vi "ThermoV_ControlSweep_NoMean_ExperimentalCode_AC_LV2017.vi"() -> ()   [LabVIEW 2017]
panel:
  in  "Operate HVpp\nOutput Timer":bool caption="Reset"
  out "modular 13":dbl
  in  "Number of seconds for \neach HVpp case state":dbl=30.0
  out "Elapsed Time (s)":dbl
  out "DC Value":dbl[](array[numeric]) format="%#.6f"
  in  "Saving Avg?":bool
  in  "Filename":path=path "trial_1.lvm"
  in  "STOP":bool
  in  "Save Waveform":bool
  out "Peak2Peak V":dbl[](array[numeric])
  out "Waveform Chart":dynamicdata(graph)
  # "AI 0:  Thermoelectric Voltage\nAI 1:  Heater Current (Voltage)\n\nAO 0:  Applied Heater Voltage"
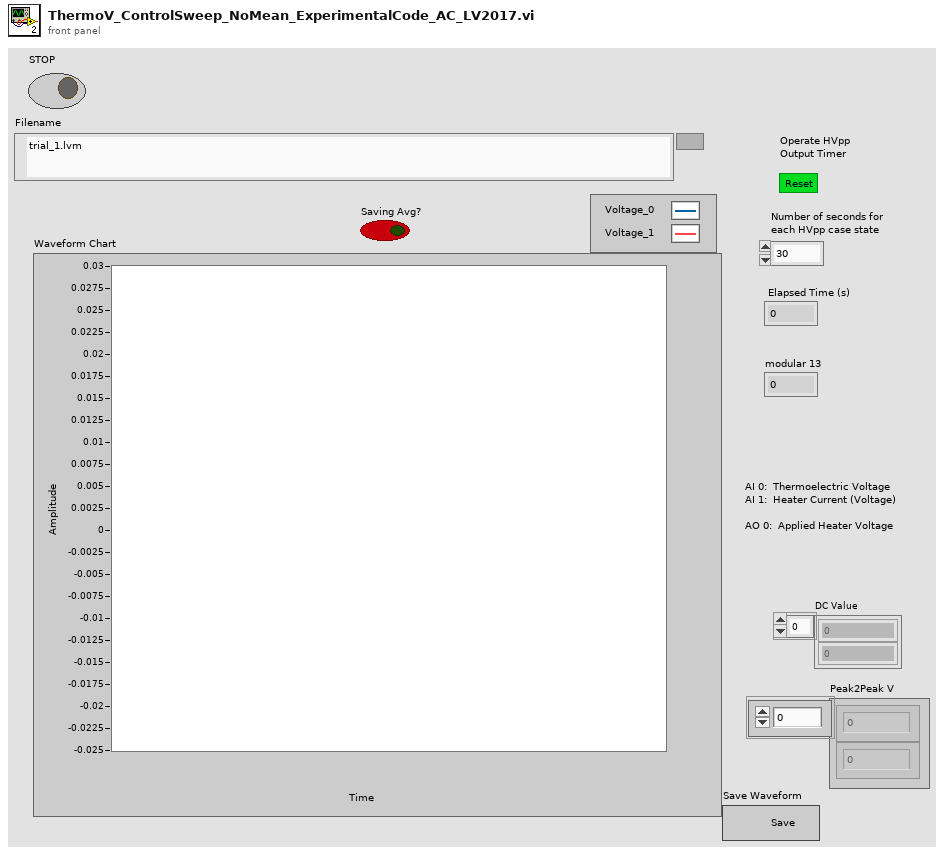
[diagram p1: front panel]
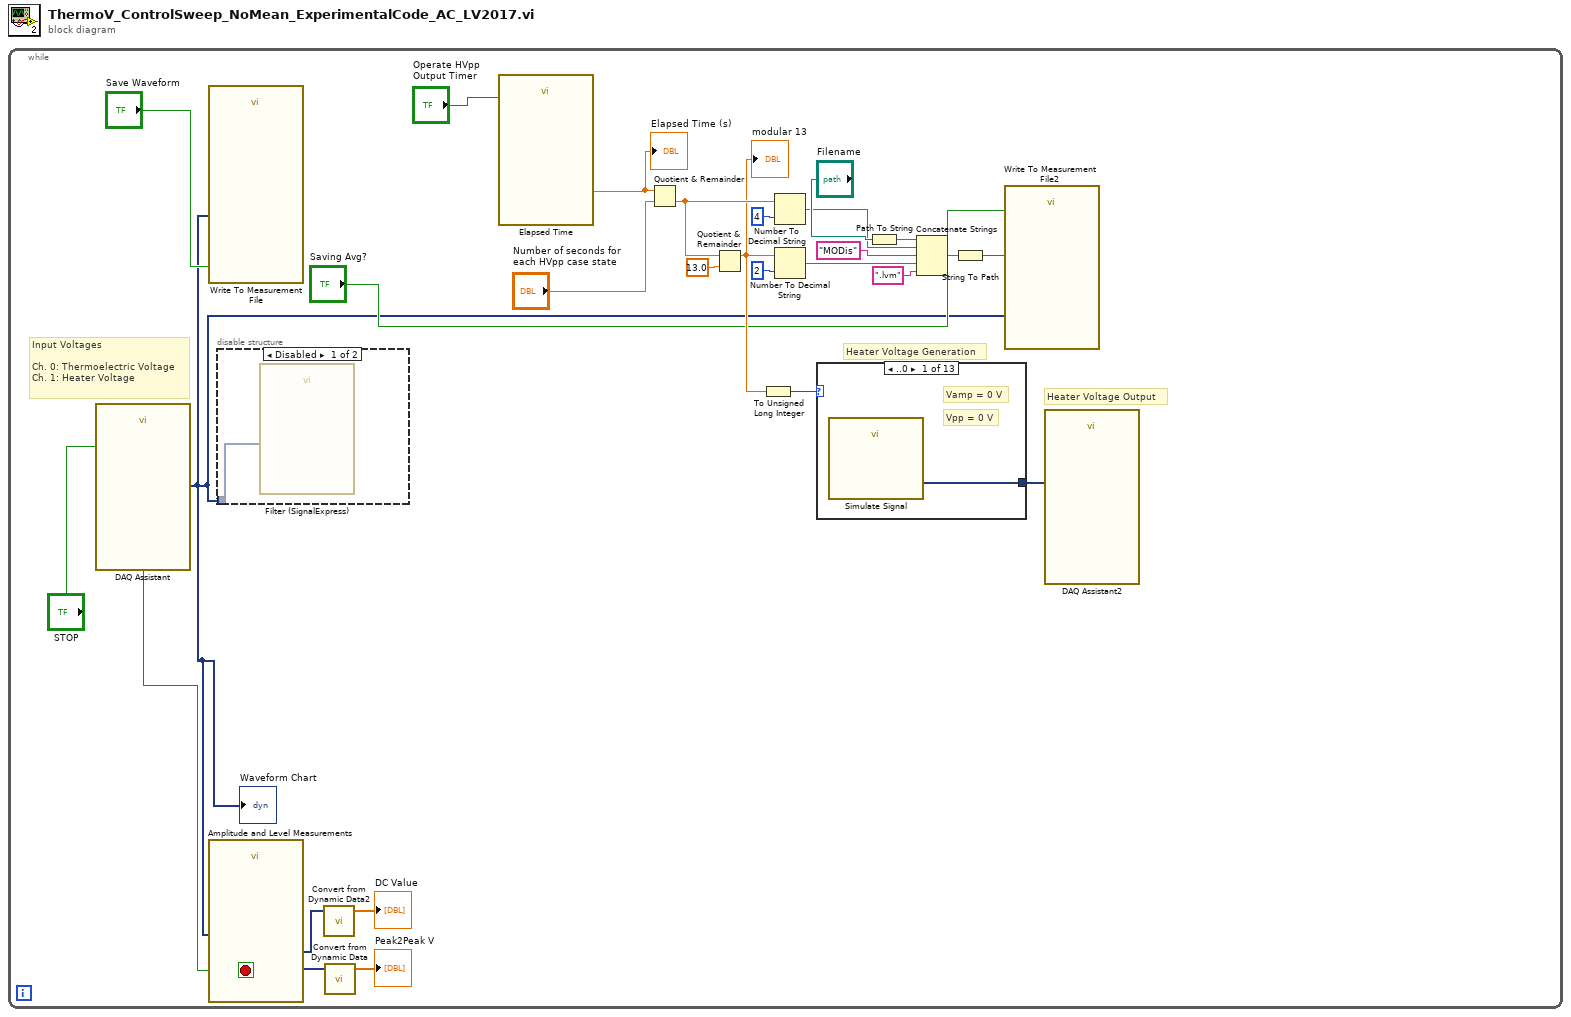
[diagram p0: block diagram]
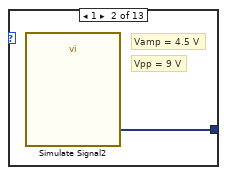
[diagram p3: hidden frame]
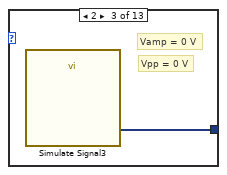
[diagram p4: hidden frame]
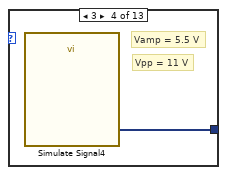
[diagram p5: hidden frame]
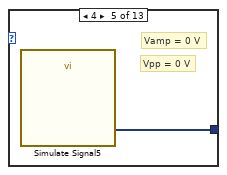
[diagram p6: hidden frame]
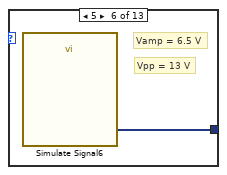
[diagram p7: hidden frame]
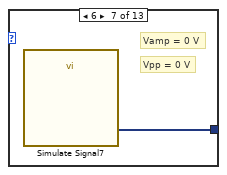
[diagram p8: hidden frame]
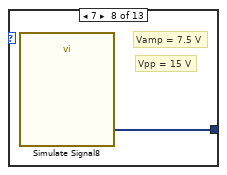
[diagram p9: hidden frame]
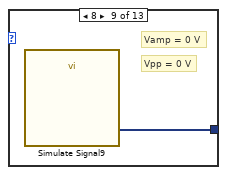
[diagram p10: hidden frame]
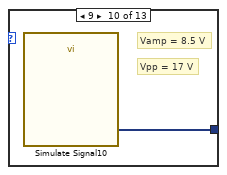
[diagram p11: hidden frame]
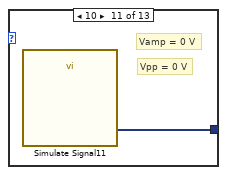
[diagram p12: hidden frame]
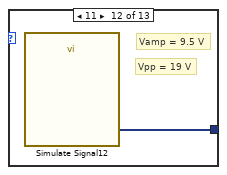
[diagram p13: hidden frame]
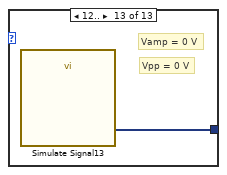
[diagram p14: hidden frame]
diagram:
  n1 = while {
    stop <- w27 stop-if-true
    # "Heater Voltage Generation"
    # "Heater Voltage Output"
    # "Input Voltages\n\nCh. 0: Thermoelectric Voltage\nCh. 1: Heater Voltage"
    n2 = call "DAQ Assistant"("stop (F)"="STOP") -> ("data"=w5:dynamicdata, "stopped"=w27:bool)  [unwired: 15 in, 2 out]
    "Waveform Chart" <- w5
    n3 = call "Write To Measurement File"("Signals"=w5, "Enable"="Save Waveform") -> ()  [unwired: 15 in, 3 out]
    n4 = call "Amplitude and Level Measurements"("Signals"=w5) -> ("Mean (DC)"=w2:dynamicdata, "Peak to Peak"=w4:dynamicdata)  [unwired: 11 in, 2 out]
    n5 = disable-structure shown="Disabled" {
      disable-tunnel: w5 -> [w28 _]
      frame Disabled {
        n6 = call "Filter (SignalExpress)"("input signal"=w28) -> ()  [unwired: 17 in, 2 out]
      }
      frame Enabled {
      }
    }
    n7 = call "Convert from Dynamic Data2"("Dynamic Data Type"=w2) -> ("Array"=→"DC Value":dbl[])  [unwired: 3 in]
    n8 = call "Convert from Dynamic Data"("Dynamic Data Type"=w4) -> ("Array"=→"Peak2Peak V":dbl[])  [unwired: 3 in]
    n9 = call "Elapsed Time"("Reset"="Operate HVpp\nOutput Timer") -> ("Elapsed Time (s)"=w22:dbl)  [unwired: 11 in, 7 out]
    "Elapsed Time (s)" <- w22
    n10 = Quotient & Remainder(x=w22, y="Number of seconds for \neach HVpp case state") -> (floor(x/y)=w14:dbl)  [unwired: 1 out]
    n11 = Quotient & Remainder(x=w14, y=13.0) -> (x-y*floor(x/y)=w9:dbl)  [unwired: 1 out]
    "modular 13" <- w9
    n12 = To Unsigned Long Integer(number=w9) -> (unsigned 32bit integer=w23:u32)
    n13 = Number To Decimal String(number=w14, width (-)=i16 4) -> (decimal integer string=w13:string)
    n14 = Number To Decimal String(number=w9, width (-)=i16 2) -> (decimal integer string=w8:string)
    n15 = case shown="..0" w23 {
      tunnel: [w29 w30 w31 w32 w33 w34 w35 w36 w37 w38 w39 w40 w41] -> w24
      frame ..0 {
        # "Vpp = 0 V"
        # "Vamp = 0 V"
        n16 = call "Simulate Signal"() -> ("DC"=w29:dynamicdata)  [unwired: 14 in, 1 out]
      }
      frame 1 {
        # "Vpp = 9 V"
        # "Vamp = 4.5 V"
        n17 = call "Simulate Signal2"() -> ("Sine"=w30:dynamicdata)  [unwired: 14 in, 1 out]
      }
      frame 2 {
        # "Vpp = 0 V"
        # "Vamp = 0 V"
        n18 = call "Simulate Signal3"() -> ("DC"=w31:dynamicdata)  [unwired: 14 in, 1 out]
      }
      frame 3 {
        # "Vpp = 11 V"
        # "Vamp = 5.5 V"
        n19 = call "Simulate Signal4"() -> ("Sine"=w32:dynamicdata)  [unwired: 14 in, 1 out]
      }
      frame 4 {
        # "Vpp = 0 V"
        # "Vamp = 0 V"
        n20 = call "Simulate Signal5"() -> ("DC"=w33:dynamicdata)  [unwired: 14 in, 1 out]
      }
      frame 5 {
        # "Vpp = 13 V"
        # "Vamp = 6.5 V"
        n21 = call "Simulate Signal6"() -> ("Sine"=w34:dynamicdata)  [unwired: 14 in, 1 out]
      }
      frame 6 {
        # "Vpp = 0 V"
        # "Vamp = 0 V"
        n22 = call "Simulate Signal7"() -> ("DC"=w35:dynamicdata)  [unwired: 14 in, 1 out]
      }
      frame 7 {
        # "Vpp = 15 V"
        # "Vamp = 7.5 V"
        n23 = call "Simulate Signal8"() -> ("Sine"=w36:dynamicdata)  [unwired: 14 in, 1 out]
      }
      frame 8 {
        # "Vpp = 0 V"
        # "Vamp = 0 V"
        n24 = call "Simulate Signal9"() -> ("DC"=w37:dynamicdata)  [unwired: 14 in, 1 out]
      }
      frame 9 {
        # "Vpp = 17 V"
        # "Vamp = 8.5 V"
        n25 = call "Simulate Signal10"() -> ("Sine"=w38:dynamicdata)  [unwired: 14 in, 1 out]
      }
      frame 10 {
        # "Vpp = 0 V"
        # "Vamp = 0 V"
        n26 = call "Simulate Signal11"() -> ("DC"=w39:dynamicdata)  [unwired: 14 in, 1 out]
      }
      frame 11 {
        # "Vpp = 19 V"
        # "Vamp = 9.5 V"
        n27 = call "Simulate Signal12"() -> ("Sine"=w40:dynamicdata)  [unwired: 14 in, 1 out]
      }
      frame 12.. {
        # "Vpp = 0 V"
        # "Vamp = 0 V"
        n28 = call "Simulate Signal13"() -> ("DC"=w41:dynamicdata)  [unwired: 14 in, 1 out]
      }
    }
    n29 = Path To String(path="Filename") -> (string=w16:string)
    n30 = Concatenate Strings(w16, w13, "MODis" ("string"), w8, ".lvm" ("string")) -> (w18:string)
    n31 = String To Path(string=w18) -> (path=w19:path)
    n32 = call "Write To Measurement File2"("Signals"=w5, "Enable"="Saving Avg?", "Filename"=w19) -> ()  [unwired: 14 in, 3 out]
    n33 = call "DAQ Assistant2"("data"=w24) -> ()  [unwired: 16 in, 3 out]
  }
